vi "OnDrop.vi"(0 "XRef":T5, 1 "State In":T1) -> (14 "Reply":T3, 15 "Fatal Error Out":T2, 16 "State Out":T1)   [LabVIEW 2015, in "Build JSON Array.xnode"]
uses:
  Build JSON Array.xnode
  <vilib>/XNodeSupport/XNodeXNodeRef.ctl
  State.ctl
  <vilib>/XNodeSupport/XNodeStringArray.ctl
  <vilib>/XNodeSupport/XNodeString.ctl
  <vilib>/XNodeSupport/XNodeErrorCluster.ctl
  <vilib>/Utility/miscctls.llb/LVPointTypeDef.ctl
  class loader.vi
  <vilib>/XNodeSupport/NI_XNodeSupport.lvlib
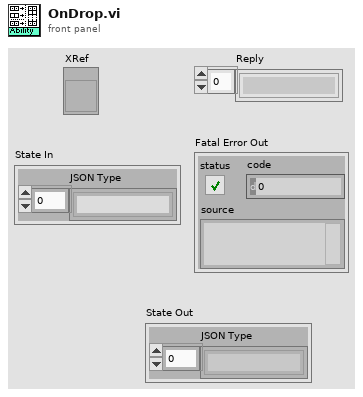
[diagram p1: front panel]
types:
  T1 = typedef "Build JSON Array.xnode/State.ctl" = cluster{"JSON Type":string[]}
  T2 = typedef "NI_XNodeSupport.lvlib/XNodeErrorCluster.ctl" = errorcluster
  T3 = typedef "NI_XNodeSupport.lvlib/XNodeStringArray.ctl" = T4[]
  T4 = typedef "NI_XNodeSupport.lvlib/XNodeString.ctl" = string
  T5 = typedef "NI_XNodeSupport.lvlib/XNodeXNodeRef.ctl" = refnum<vi>
  T6 = typedef "LVPointTypeDef.ctl" = cluster{"Horizontal":i16, "Vertical":i16}
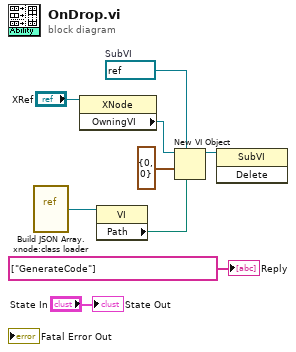
[diagram p0: block diagram]
diagram:
  w6 = refnum<vi> refnum  # SubVI
  n1 = vi-ref "Build JSON Array.xnode:class loader.vi"() -> (w3:refnum<vi>)
  n2 = property class="XNode"(reference="XRef") -> ("OwningVI"=w7:refnum<vi>)  [unwired: 1 in, 2 out]
  n3 = property class="VI"(reference=w3) -> ("Path"=w2:path)  [unwired: 1 in, 2 out]
  n4 = New VI Object(vi object class=w6, owner refnum=w7, position/next to=T6 {"Horizontal"=0, "Vertical"=0} ("location"), 6:w2) -> (object refnum=w4:refnum<vi>)  [unwired: 4 in, 1 out]
  n5 = invoke class="SubVI" method="Delete"(reference=w4) -> ()  [unwired: 2 in, 3 out]
  "Reply" <- T3 ["GenerateCode"] ("Reply")
  "State Out" <- "State In"
